vi "NI9188 Producer.vi"(7 "Physical Channels":string, 8 "error in":errorcluster, 9 "Samples per Channel":i32=100, 10 "Sample Rate":dbl=100000.0, 11 "Data Queue":refnum<queue>) -> (0 "error out":errorcluster, 2 "Restart":bool)   [LabVIEW 2013]
uses:
  <vilib>/DAQmx/create/channels.llb/DAQmx Create Channel (AI-Voltage-Basic).vi
  <vilib>/DAQmx/configure/timing.llb/DAQmx Timing (Sample Clock).vi
  <vilib>/DAQmx/create/channels.llb/DAQmx Create Channel (CO-Pulse Generation-Frequency).vi
  <vilib>/DAQmx/configure/timing.llb/DAQmx Timing (Implicit).vi
  <vilib>/DAQmx/configure/trigger.llb/DAQmx Start Trigger (Digital Edge).vi
  SCM Breakdown Locator/UDP Heartbeat Globals.vi
  Execution Control Global.vi
  <vilib>/DAQmx/read.llb/DAQmx Read (Analog 1D Wfm NChan NSamp).vi
  <resource>/objmgr/daqmx.rc
panel:
  out "name":string
  in  "Remote UDP Port":u16=31416
  out "Spark Flag Synch\nLoop Time (ms)":u32
  in  "Stop":bool
  out "Spark!":bool
  in  "Local UDP Port":u16=31417
  in  "Synch Delay (ms)":u16=50
  out "ms since last read":u32
  out "Waveform Graph":waveform(dbl)[](graph)
  out "Actual Sample Rate":dbl=1000.0 format="%0.2f"
  # "Acquired Data"
  # "Settings"
  # "Logging Settings"
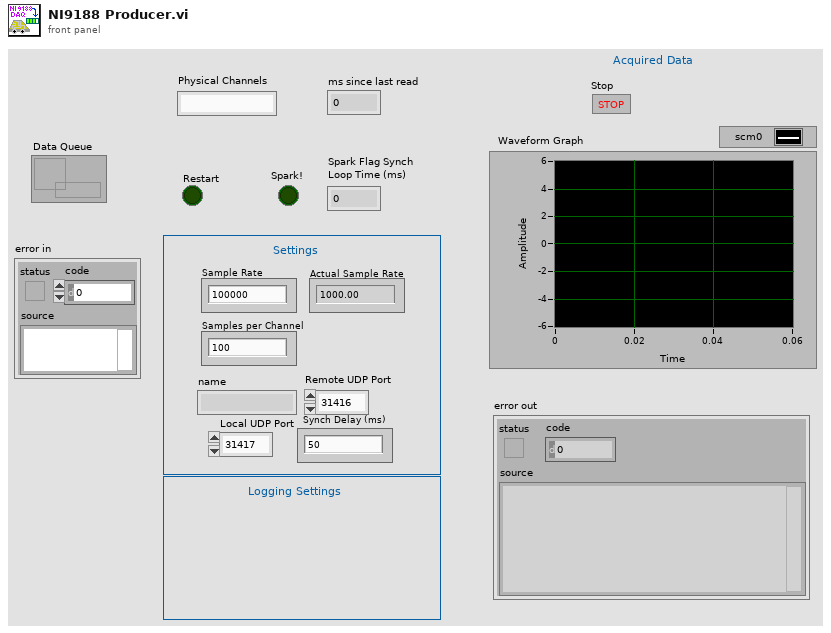
[diagram p1: front panel]
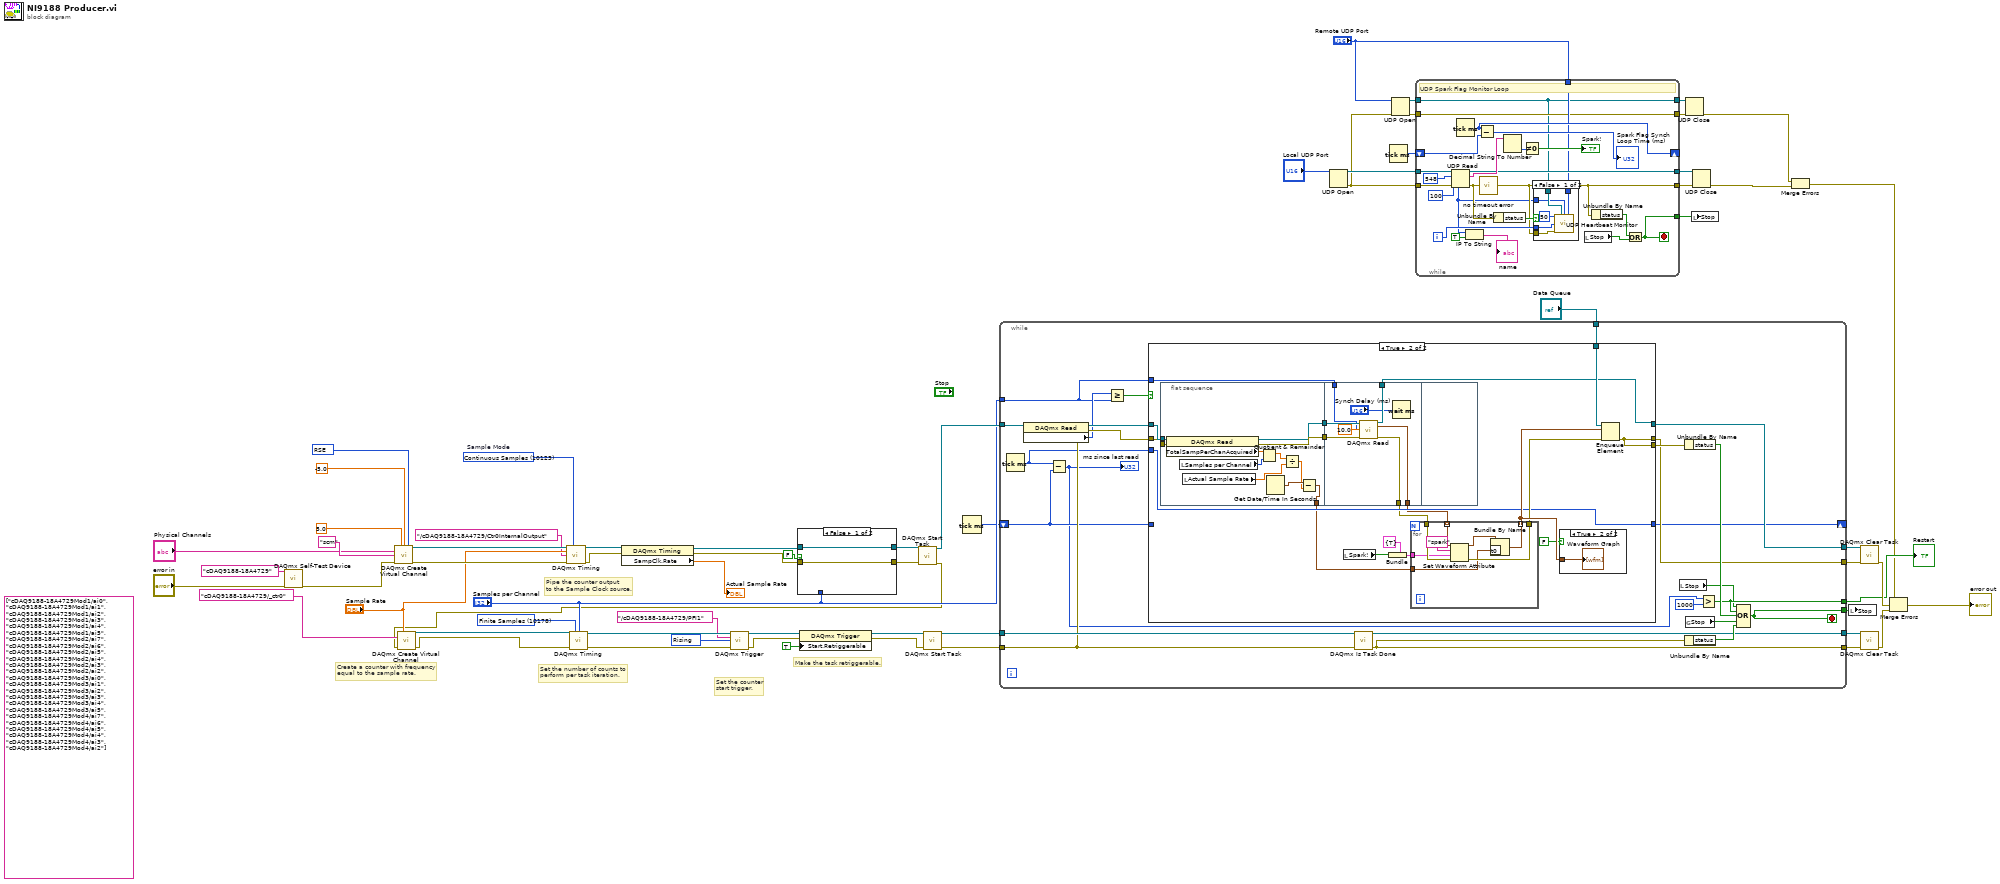
[diagram p0: block diagram]
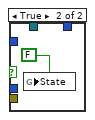
[diagram p2: hidden frame]
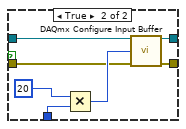
[diagram p3: hidden frame]
diagram:
  w33 = 10280 items=["Rising"=10280, "Falling"=10171] ("edge")
  w59 = 10083 items=["default"=-1, "RSE"=10083, "NRSE"=10078, "Differential"=10106, "Pseudodifferential"=12529] ("Terminal Configuration")
  w53 = 10178 items=["Finite Samples"=10178, "Continuous Samples"=10123, "Hardware Timed Single Point"=12522] ("sample mode")
  (unwired) tag[] ["cDAQ9188-18A4729Mod1/ai0", "cDAQ9188-18A4729Mod1/ai1", "cDAQ9188-18A4729Mod1/ai2", "cDAQ9188-18A4729Mod1/ai3", "cDAQ9188-18A4729Mod1/ai4", "cDAQ9188-18A4729Mod1/ai5", "cDAQ9188-18A4729Mod2/ai7", "cDAQ9188-18A4729Mod2/ai6", "cDAQ9188-18A4729Mod2/ai5", "cDAQ9188-18A4729Mod2/ai4", "cDAQ9188-18A4729Mod2/ai3", "cDAQ9188-18A4729Mod2/ai2", "cDAQ9188-18A4729Mod3/ai0", "cDAQ9188-18A4729Mod3/ai1", "cDAQ9188-18A4729Mod3/ai2", "cDAQ9188-18A4729Mod3/ai3", "cDAQ9188-18A4729Mod3/ai4", "cDAQ9188-18A4729Mod3/ai5", "cDAQ9188-18A4729Mod4/ai7", "cDAQ9188-18A4729Mod4/ai6", "cDAQ9188-18A4729Mod4/ai5", "cDAQ9188-18A4729Mod4/ai4", "cDAQ9188-18A4729Mod4/ai3", "cDAQ9188-18A4729Mod4/ai2"]
  w63 = 10123 items=["Finite Samples"=10178, "Continuous Samples"=10123, "Hardware Timed Single Point"=12522]  # Sample Mode
  # "Set the counter\nstart trigger."
  # "Make the task retriggerable."
  # "Set the number of counts to\nperform per task iteration."
  # "Pipe the counter output\nto the Sample Clock source."
  # "Create a counter with frequency\nequal to the sample rate."
  n1 = call <vilib>:"DAQmx Self-Test Device.vi"("device in"=tag "cDAQ9188-18A4729", "error in"="error in") -> ("error out"=w2:errorcluster)  [unwired: 13 in]
  n2 = call-poly <vilib>:"DAQmx Create Virtual Channel.vi"("maximum value"=5.0 ("Max Voltage"), "minimum value"=-5.0 ("Min Voltage"), "input terminal configuration"=w59, "physical channels"="Physical Channels", "name to assign"="scm", "error in"=w2) -> ("task out"=w61:refnum<k21>, "error out"=w62:errorcluster)  [unwired: 8 in]
  n3 = call-poly <vilib>:"DAQmx Timing.vi"("task/channels in"=w61, "sample mode"=w63, "rate"="Sample Rate", "source"=tag "/cDAQ9188-18A4729/Ctr0InternalOutput" ("CO.Pulse.Term"), "error in"=w62) -> ("task out"=w65:refnum<k21>, "error out"=w64:errorcluster)  [unwired: 9 in]
  n4 = property class="DAQmx Timing"(reference=w65, error in=w64) -> (reference out=w4:refnum<k21>, error out=w3:errorcluster, "SampClk.Rate"=→"Actual Sample Rate":dbl)
  n5 = case shown="False" FALSE {
    tunnel: w4 -> [w67 w73]
    tunnel: w3 -> [w66 w72]
    tunnel: [w67 w71] -> w38
    tunnel: [w66 w70] -> w37
    tunnel: "Samples per Channel" -> [_ w68]
    frame False {
    }
    frame True {
      n6 = Multiply(x=u32 20, y=w68) -> (x*y=w74:u32)
      n7 = call <vilib>:"DAQmx Configure Input Buffer.vi"("task/channels in"=w73, "buffer size (in samples per channel)"=w74, "error in"=w72) -> ("task out"=w71:refnum<k21>, "error out"=w70:errorcluster)  [unwired: 11 in]
    }
  }
  n8 = call <vilib>:"DAQmx Start Task.vi"("task/channels in"=w38, "error in"=w37) -> ("task out"=w45:refnum<k21>, "error out"=w28:errorcluster)  [unwired: 12 in]
  n9 = call-poly <vilib>:"DAQmx Create Virtual Channel.vi"("frequency"="Sample Rate", "counter"=tag "cDAQ9188-18A4729/_ctr0" ("Counter*"), "error in"=w28) -> ("task out"=w30:refnum<k21>, "error out"=w29:errorcluster)  [unwired: 11 in]
  n10 = call-poly <vilib>:"DAQmx Timing.vi"("task/channels in"=w30, "sample mode"=w53, "samples per channel"="Samples per Channel", "error in"=w29) -> ("task out"=w51:refnum<k21>, "error out"=w50:errorcluster)  [unwired: 10 in]
  n11 = call-poly <vilib>:"DAQmx Trigger.vi"("task/channels in"=w51, "source"=tag "/cDAQ9188-18A4729/PFI1" ("Trigger Source"), "edge"=w33, "error in"=w50) -> ("task out"=w49:refnum<k21>, "error out"=w48:errorcluster)  [unwired: 10 in]
  n12 = property class="DAQmx Trigger"(reference=w49, error in=w48, "Start.Retriggerable"=TRUE) -> (reference out=w44:refnum<k21>, error out=w43:errorcluster)
  n13 = call <vilib>:"DAQmx Start Task.vi"("task/channels in"=w44, "error in"=w43) -> ("task out"=w42:refnum<k21>, "error out"=w41:errorcluster)  [unwired: 12 in]
  n14 = Tick Count (ms)() -> (millisecond timer value=w27:u32)
  n15 = while {
    tunnel: "Samples per Channel" -> [w77]
    tunnel: w45 -> [w90]
    tunnel: [w95] -> w55
    tunnel: [w94] -> w54
    tunnel: w42 -> [w97]
    tunnel: w41 -> [w87]
    tunnel: [w93] -> w40
    tunnel: [w92] -> w39
    tunnel: "Data Queue" -> [w84]
    shift-right: [w81] -> _
    shift-left: w27 -> [w83]
    tunnel: [w79] -> w23
    tunnel: [w75] -> w15
    stop <- w75 stop-if-true
    n16 = Tick Count (ms)() -> (millisecond timer value=w82:u32)
    n17 = property class="DAQmx Read"(reference=w90, error in=w87) -> (reference out=w89:refnum<k21>, error out=w88:errorcluster, "Status:Available Samples Per Channel"=w85:u32)
    n18 = Subtract(x=w82, y=w83) -> (x-y=w78:u32)
    "ms since last read" <- w78
    n19 = Greater Or Equal?(x=w85, y=w77) -> (x >= y?=w86:bool)
    n20 = case shown="True" w86 {
      tunnel: [w100 w117] -> w98
      tunnel: w89 -> [w101 w120]
      tunnel: w88 -> [w100 w119]
      tunnel: [w101 w104] -> w95
      tunnel: [w100 w117] -> w94
      tunnel: w84 -> [_ w118]
      tunnel: [w102 w114] -> w81
      tunnel: w83 -> [w102 _]
      tunnel: w82 -> [_ w114]
      tunnel: w77 -> [_ w108]
      frame False {
      }
      frame True {
        n21 = flat-sequence {
          tunnel: w119 -> [w130]
          tunnel: w120 -> [w131]
          tunnel: [w128] -> w110
          tunnel: [w129] -> w109
          tunnel: [w126] -> w107
          tunnel: w110 -> [w139]
          tunnel: w109 -> [w138]
          tunnel: w108 -> [w136]
          tunnel: [w135] -> w106
          tunnel: [w134] -> w105
          tunnel: [w133] -> w104
          frame #0 {
            n22 = property class="DAQmx Read"(reference=w131, error in=w130) -> (reference out=w128:refnum<k21>, error out=w129:errorcluster, "TotalSampPerChanAcquired"=w124:dbl)
            n23 = local read "Samples per Channel"() -> (w125:i32)
            n24 = local read "Actual Sample Rate"() -> (w122:dbl)
            n25 = Quotient & Remainder(x=w124, y=w125) -> (x-y*floor(x/y)=w123:dbl)  [unwired: 1 out]
            n26 = Get Date/Time In Seconds() -> (seconds since 1Jan1904=w127:timestamp)
            n27 = Divide(x=w123, y=w122) -> (x/y=w121:dbl)
            n28 = Subtract(x=w127, y=w121) -> (x-y=w126:timestamp)
          }
          frame #1 {
            n29 = call-poly <vilib>:"DAQmx Read.vi"("task/channels in"=w139, "number of samples per channel"=w136, "timeout"=10.0, "error in"=w138) -> ("task out"=w133:refnum<k21>, "data"=w134:waveform(dbl)[], "error out"=w135:errorcluster)  [unwired: 9 in]
            n30 = Wait (ms)(milliseconds to wait="Synch Delay (ms)") -> ()  [unwired: 1 out]
          }
          frame #2 {
          }
        }
        n31 = local read "Spark!"() -> (w103:bool)
        n32 = Bundle(cluster=cluster{bool} {TRUE} ("value"), w103) -> (w111:cluster{bool})
        n33 = for {
          tunnel: w105 -> [w147] mode=indexing
          tunnel: [w141] -> w116 mode=indexing
          tunnel: w106 -> [w146]
          tunnel: [w145] -> w115
          tunnel: w111 -> [w143]
          tunnel: w107 -> [w140]
          n34 = Set Waveform Attribute(4:w146, 5:w143, 6:"spark" ("name"), 7:w147) -> (0:w145:errorcluster, 3:w142:waveform(dbl))  [unwired: 1 out]
          n35 = Bundle By Name(cluster=w142, "t0"=w140) -> (w141:waveform(dbl))
        }
        n36 = case shown="True" FALSE {
          tunnel: w116 -> [_ w148]
          frame False {
          }
          frame True {
            "Waveform Graph" <- w148
          }
        }
        n37 = Enqueue Element(queue=w118, element=w116, error in (no error)=w115) -> (error out=w117:errorcluster)  [unwired: 1 in, 2 out]
      }
    }
    n38 = call <vilib>:"DAQmx Is Task Done.vi"("task/channels in"=w97, "error in"=w87) -> ("task out"=w93:refnum<k21>, "error out"=w92:errorcluster)  [unwired: 11 in, 1 out]
    n39 = local read "Stop"() -> (w76:bool)
    n40 = Unbundle By Name(w98) -> ("status"=w99:bool)
    n41 = Unbundle By Name(w92) -> ("status"=w96:bool)
    n42 = global read "Execution Control Global.vi" "Stop"() -> (w91:bool)
    n43 = Greater?(x=w78, y=u32 1000) -> (0:w79:bool)
    n44 = Compound Arithmetic op=OR(w76, w79, w99, w91, w96) -> (w75:bool)
  }
  "Restart" <- w23
  n45 = UDP Open(11:"Local UDP Port") -> (port=w20:refnum<k16>, 0:w11:errorcluster)  [unwired: 4 in, 1 out]
  n46 = Tick Count (ms)() -> (millisecond timer value=w14:u32)
  n47 = UDP Open(8:w11, 11:"Remote UDP Port") -> (port=w12:refnum<k16>, 0:w10:errorcluster)  [unwired: 3 in, 1 out]
  n48 = while {
    tunnel: w20 -> [w171]
    tunnel: w11 -> [w170]
    tunnel: [w156] -> w19
    tunnel: [w155] -> w18
    tunnel: [w166] -> w16
    shift-right: [w161] -> _
    shift-left: w14 -> [w163]
    tunnel: "Remote UDP Port" -> [w154]
    tunnel: w12 -> [w152]
    tunnel: [w153] -> w9
    tunnel: w10 -> [w153]
    tunnel: [w152] -> w8
    i -> [w158]
    stop <- w166 stop-if-true
    # "UDP Spark Flag Monitor Loop"
    n49 = UDP Read(connection ID=w171, max size (548)=548 ("max bytes/read"), timeout ms (25000)=100, 8:w170) -> (data out=w172:string, error out=w159:errorcluster, 3:w155:refnum<k16>, 6:w151:u32)  [unwired: 1 out]
    n50 = Tick Count (ms)() -> (millisecond timer value=w161:u32)
    n51 = IP To String(1:TRUE ("dot notation? (F)"), 2:w151) -> (0:→"name":string)
    n52 = Subtract(x=w161, y=w163) -> (x-y=→"Spark Flag Synch\nLoop Time (ms)":u32)
    n53 = call "no timeout error.vi"("error in (no error)"=w159) -> ("error out"=w156:errorcluster)
    n54 = Unbundle By Name(w159) -> ("status"=w157:bool)
    n55 = Decimal String To Number(string=w172) -> (number=w165:i32)  [unwired: 2 in, 1 out]
    n56 = Not Equal To 0?(x=w165) -> (x != 0?=→"Spark!":bool)
    n57 = case shown="False" w157 {
      tunnel: w158 -> [w177 _]
      tunnel: w156 -> [w176 _]
      tunnel: w152 -> [w175 _]
      tunnel: w154 -> [w174 _]
      tunnel: w151 -> [w173 _]
      frame False {
        n58 = call "UDP Heartbeat Monitor.vi"("Interval Length"=50, "connection ID"=w175, "Remote UDP Address"=w173, "Remote UDP Port"=w174, "Count"=w177, "error in (no error)"=w176) -> ()  [unwired: 9 in, 1 out]
      }
      frame True {
        n59 = global write "UDP Heartbeat Globals.vi" "State"(FALSE) -> ()
      }
    }
    n60 = local read "Stop"() -> (w167:bool)
    n61 = Unbundle By Name(w156) -> ("status"=w168:bool)
    n62 = Or(x=w168, y=w167) -> (x .or. y?=w166:bool)
  }
  n63 = UDP Close(connection ID=w8, 8:w9) -> (error out=w6:errorcluster)  [unwired: 1 out]
  n64 = local write "Stop"(w16) -> ()
  n65 = UDP Close(connection ID=w18, 8:w19) -> (error out=w5:errorcluster)  [unwired: 1 out]
  n66 = Merge Errors(w6, w5) -> (w7:errorcluster)
  n67 = local write "Stop"(w15) -> ()
  n68 = call <vilib>:"DAQmx Clear Task.vi"("task in"=w55, "error in"=w54) -> ("error out"=w31:errorcluster)  [unwired: 13 in]
  n69 = call <vilib>:"DAQmx Clear Task.vi"("task in"=w40, "error in"=w39) -> ("error out"=w32:errorcluster)  [unwired: 13 in]
  n70 = Merge Errors(w7, w31, w32) -> (→"error out":errorcluster)
